vi "Sub01_01_BorderFinder.vi"(8 "error in (no error)":errorcluster, 10 "Border":T1, 11 "image data":T2) -> (0 "error out":errorcluster, 1 "Cmin":i32, 2 "Lmax":u32, 3 "Lmin":i32, 4 "Cmax":u32)   [LabVIEW 2019]
uses:
  <vilib>/picture/picture.llb/imagedata.ctl
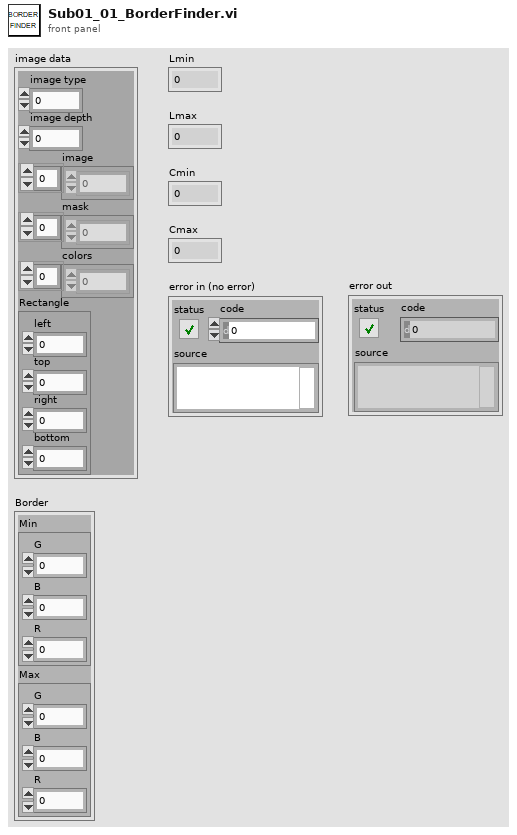
[diagram p1: front panel]
types:
  T1 = cluster{"Min":cluster{"G":u32, "B":u32, "R":u32}, "Max":cluster{"G":u32, "B":u32, "R":u32}}
  T2 = typedef "imagedata.ctl" = cluster{"image type":i32, "image depth":i32, "image":u8[], "mask":u8[], "colors":u32[], "Rectangle":cluster{"left":i16, "top":i16, "right":i16, "bottom":i16}}
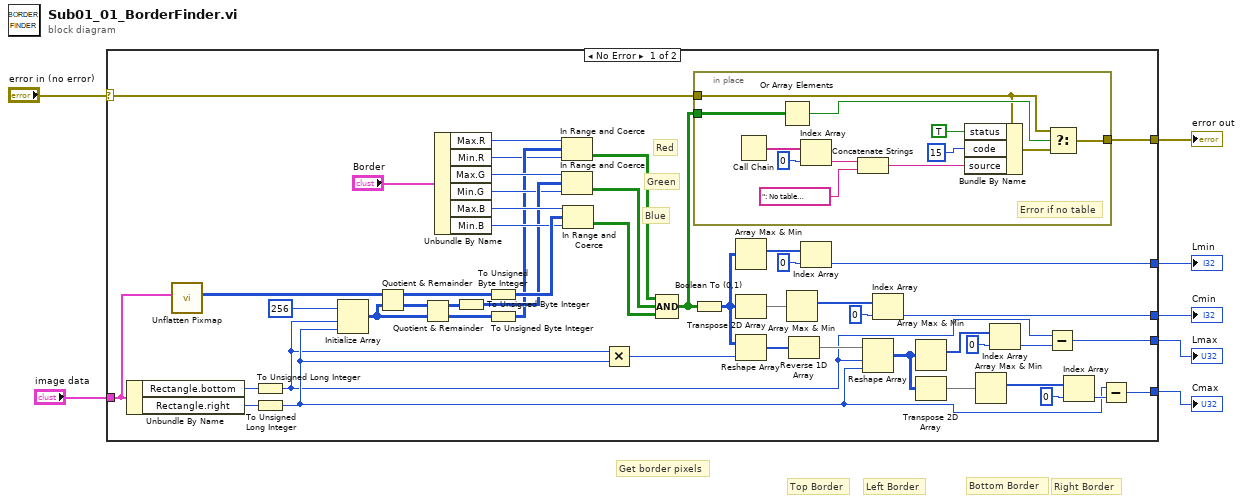
[diagram p0: block diagram]
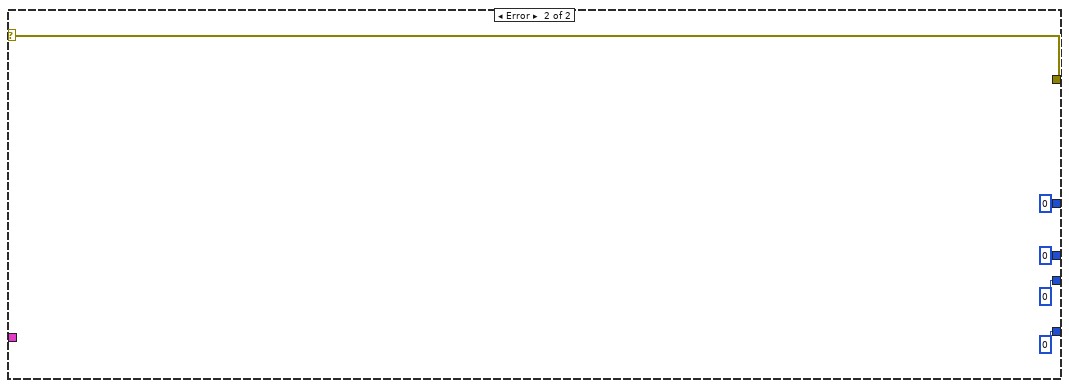
[diagram p2: hidden frame]
diagram:
  # "Get border pixels"
  # "Right Border"
  # "Bottom Border"
  # "Left Border"
  # "Top Border"
  n1 = case shown="No Error" "error in (no error)" {
    selector: "error in (no error)" -> [w53 w69]
    tunnel: [w12 u32 0] -> w7
    tunnel: [w13 u32 0] -> w6
    tunnel: [w11 0] -> w5
    tunnel: [w10 0] -> w4
    tunnel: [w54 w69] -> w3
    tunnel: "image data" -> [w52 _]
    frame No Error {
      # "Red"
      # "Green"
      # "Blue"
      n2 = Unbundle By Name(w52) -> ("Rectangle.bottom"=w55:i16, "Rectangle.right"=w56:i16)
      n3 = call <vilib>:"Unflatten Pixmap.vi"("image data"=w52) -> ("24-bit pixmap"=w33:u32[][])  [unwired: 4 in, 6 out]
      n4 = To Unsigned Long Integer(number=w55) -> (unsigned 32bit integer=w8:u32)
      n5 = To Unsigned Long Integer(number=w56) -> (unsigned 32bit integer=w9:u32)
      n6 = Initialize Array(u32 256 ("element"), w8, w9) -> (w34:u32[][])
      n7 = Quotient & Remainder(x=w33, y=w34) -> (x-y*floor(x/y)=w38:u32[][], floor(x/y)=w35:u32[][])
      n8 = Quotient & Remainder(x=w35, y=w34) -> (x-y*floor(x/y)=w36:u32[][], floor(x/y)=w37:u32[][])
      n9 = Unbundle By Name("Border") -> ("Max.R"=w42:u32, "Min.R"=w40:u32, "Max.G"=w45:u32, "Min.G"=w43:u32, "Max.B"=w48:u32, "Min.B"=w46:u32)
      n10 = To Unsigned Byte Integer(number=w36) -> (unsigned 8bit integer=w44:u8[][])
      n11 = To Unsigned Byte Integer(number=w38) -> (unsigned 8bit integer=w47:u8[][])
      n12 = To Unsigned Byte Integer(number=w37) -> (unsigned 8bit integer=w41:u8[][])
      n13 = In Range and Coerce(upper limit=w42, x=w41, lower limit=w40) -> (In Range?=w49:bool[][])  [unwired: 1 out]
      n14 = In Range and Coerce(upper limit=w45, x=w44, lower limit=w43) -> (In Range?=w50:bool[][])  [unwired: 1 out]
      n15 = In Range and Coerce(upper limit=w48, x=w47, lower limit=w46) -> (In Range?=w51:bool[][])  [unwired: 1 out]
      n16 = Multiply(x=w8, y=w9) -> (x*y=w14:u32)
      n17 = Compound Arithmetic op=AND(w49, w50, w51) -> (w31:bool[][])
      n18 = in-place {
        in-place-border: [w65] -> w54
        in-place-border: w53 -> [w63]
        in-place-border: w31 -> [w57]
        # "Error if no table"
        n19 = Call Chain() -> (call chain=w62:string[])
        n20 = Or Array Elements(Boolean array=w57) -> (logical OR=w66:bool)
        n21 = Index Array(array=w62, index=0) -> (element=w60:string)
        n22 = Concatenate Strings(w60, ": No table detected" ("source")) -> (w58:string)
        n23 = Bundle By Name(cluster=w63, "status"=TRUE, "code"=15, "source"=w58) -> (w64:errorcluster)
        n24 = Select(t=w63, s=w66, f=w64) -> (s? t:f=w65:errorcluster)
      }
      n25 = Boolean To (0,1)(Boolean=w31) -> (0, 1=w15:i16[][])
      n26 = Array Max & Min(array=w15) -> (max index (indices)=w25:i32[])  [unwired: 3 out]
      n27 = Transpose 2D Array(2D array=w15) -> (transposed array=w29:i16[][])
      n28 = Reshape Array(w15, w14) -> (w27:i16[])
      n29 = Array Max & Min(array=w29) -> (max index (indices)=w24:i32[])  [unwired: 3 out]
      n30 = Reverse 1D Array(array=w27) -> (reversed array=w30:i16[])
      n31 = Index Array(array=w25, index=0) -> (element=w10:i32)
      n32 = Reshape Array(w30, w8, w9) -> (w26:i16[][])
      n33 = Index Array(array=w24, index=0) -> (element=w11:i32)
      n34 = Array Max & Min(array=w26) -> (max index (indices)=w22:i32[])  [unwired: 3 out]
      n35 = Transpose 2D Array(2D array=w26) -> (transposed array=w28:i16[][])
      n36 = Array Max & Min(array=w28) -> (max index (indices)=w23:i32[])  [unwired: 3 out]
      n37 = Index Array(array=w22, index=0) -> (element=w21:i32)
      n38 = Subtract(x=w8, y=w21) -> (x-y=w13:u32)
      n39 = Index Array(array=w23, index=0) -> (element=w20:i32)
      n40 = Subtract(x=w9, y=w20) -> (x-y=w12:u32)
    }
    frame Error {
    }
  }
  "Cmax" <- w7
  "Lmax" <- w6
  "Cmin" <- w5
  "Lmin" <- w4
  "error out" <- w3
